vi "Get 40MHz Looprate.vi"() -> (1 "Looprate":sgl)   [LabVIEW 2020]
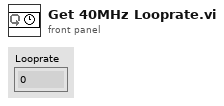
[diagram p1: front panel]
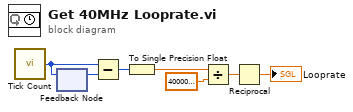
[diagram p0: block diagram]
diagram:
  n1 = call "Tick Count"() -> ("Tick Count(Ticks)"=w5:u32)
  n2 = feedback #1() -> (w6:u32)  [unwired: 1 in]
  n3 = feedback-in #1(w5) -> ()
  n4 = Subtract(x=w5, y=w6) -> (x-y=w7:u32)
  n5 = To Single Precision Float(number=w7) -> (single precision float=w1:sgl)
  n6 = Divide(x=w1, y=sgl 40000000.0) -> (x/y=w3:sgl)
  n7 = Reciprocal(x=w3) -> (1/x=→"Looprate":sgl)
